vi "Get Device Property.vi"(0 "Session Handle in":T1, 7 "property":refnum<k21>, 11 "error in (no error)":errorcluster) -> (4 "Session Handle out":T1, 6 "property value":bool, 15 "error out":errorcluster)   [LabVIEW 2015, in "SLSC Switch.lvlib" / "SLSC Session.lvclass"]
uses:
  SLSC Session.lvclass
  Typedefs/Session Handle.ctl
  SLSC Session.lvclass/SLSC Session.ctl
  <vilib>/SLSC/Get Device Property (Bool).vi
  <vilib>/SLSC/SLSC.lvlib
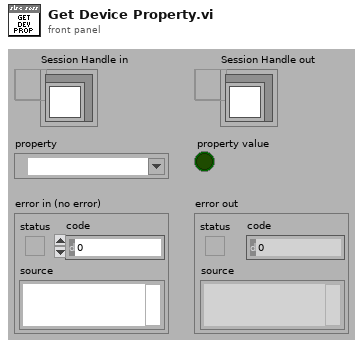
[diagram p1: front panel]
types:
  T1 = typedef "SLSC Switch.lvlib/SLSC Session.lvclass/Session Handle.ctl" = refnum<data-value>
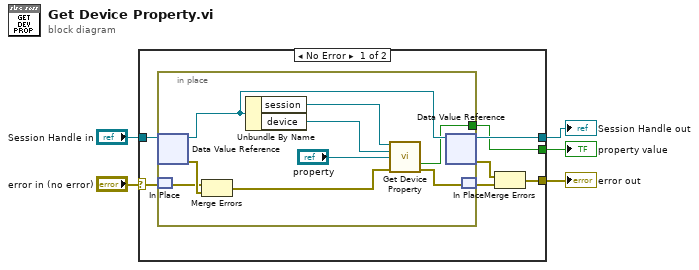
[diagram p0: block diagram]
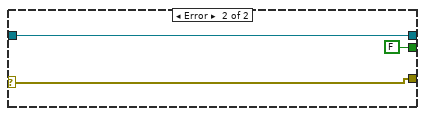
[diagram p2: hidden frame]
diagram:
  n1 = case shown="No Error" "error in (no error)" {
    selector: "error in (no error)" -> [w7 w23]
    tunnel: "Session Handle in" -> [w12 w24]
    tunnel: [w11 w24] -> w4
    tunnel: [w8 w23] -> w3
    tunnel: [w6 FALSE ("property value")] -> w1
    frame No Error {
      n2 = in-place {
        in-place-border: [w14] -> w6
        n3 = in-place-dvr #1(w12) -> (w19:refnum<class "SLSC Session.lvclass">, w21:errorcluster)
        n4 = in-place-match #2(w7) -> (w20:errorcluster)
        n5 = Merge Errors(w20, w21) -> (w17:errorcluster)
        n6 = Unbundle By Name(w19) -> ("session"=w18:refnum<k21>, "device"=w13:refnum<k21>)
        n7 = call-poly <vilib>:"Get Device Property.vi"("session in"=w18, "devices"=w13, "property"="property", "error in (no error)"=w17) -> ("property value"=w14:bool, "error out"=w16:errorcluster)  [unwired: 9 in, 1 out]
        n8 = in-place-dvr #1(w19) -> (w11:T1, w9:errorcluster)
        n9 = in-place-match #2(w16) -> (w10:errorcluster)
      }
      n10 = Merge Errors(w9, w10) -> (w8:errorcluster)
    }
    frame Error {
    }
  }
  "Session Handle out" <- w4
  "error out" <- w3
  "property value" <- w1
